vi "Module Invert Settings.vi"(7 "Keep Velocity":bool, 11 "Setting":T1 {"Angle" scale format="%.3f"; "Velocity" scale=-1.0..1.0 scale format="%.1f"}) -> (3 "Inverted Setting Out":T1 {"Angle" scale format="%.3f"; "Velocity" scale=-1.0..1.0 scale format="%.1f"})   [LabVIEW 2020, in "SwerveDrive_ACT.lvlib"]
uses:
  SwerveDrive_ACT.lvlib
  Shared Code/TypeDefs/Cluster_Module Velocity-Direction-Rotations.ctl
  Shared Code/TypeDefs/Level_Velocity plus-minus 1.ctl
  Shared Code/TypeDefs/Dial_Compase heading unit circle CCW positive.ctl
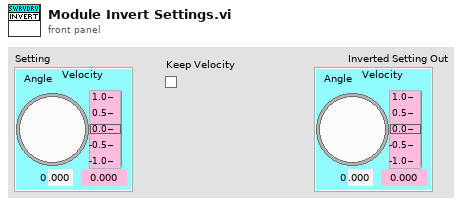
[diagram p1: front panel]
types:
  T1 = typedef "Cluster_Module Velocity-Direction-Rotations.ctl" = cluster{"Velocity":T2, "Angle":T3, "Rotations Count":dbl}
  T2 = typedef "Level_Velocity plus-minus 1.ctl" = dbl
  T3 = typedef "Dial_Compase heading unit circle CCW positive.ctl" = dbl
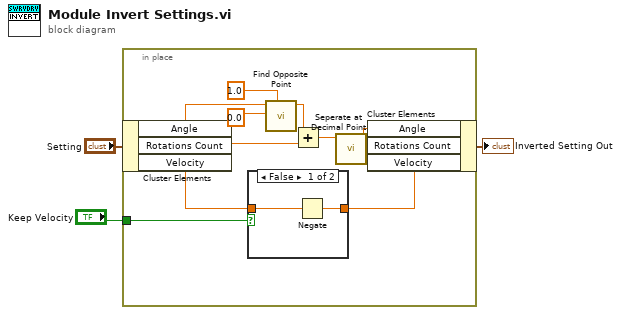
[diagram p0: block diagram]
diagram:
  n1 = in-place {
    in-place-border: "Keep Velocity" -> [w7]
    n2 = in-place-cluster #1("Setting") -> ("Angle"=w12:T3, "Rotations Count"=w10:dbl, "Velocity"=w8:T2)
    n3 = case shown="False" w7 {
      tunnel: [w16 w17] -> w9
      tunnel: w8 -> [w15 w17]
      frame False {
        n4 = Negate(x=w15) -> (-x=w16:T2)
      }
      frame True {
      }
    }
    n5 = call "Find Opposite Point.vi"("Circle Max Value"=1.0, "Circle Min Value"=0.0 ("Circle Max Value"), "Position To invert"=w12) -> ("Opposite Point Out"=w11:dbl)  [unwired: 8 in]
    n6 = Add(x=w11, y=w10) -> (x+y=w6:dbl)
    n7 = call "Seperate at Decimal Point.vi"("Rotations"=w6) -> ("Rotations"=w4:dbl, "Angle"=w5:T3)  [unwired: 9 in]
    n8 = in-place-cluster #1("Angle"=w5, "Rotations Count"=w4, "Velocity"=w9) -> (→"Inverted Setting Out":T1)
  }
